vi "LabVIEW FPGA Advanced Interface Tools Installer.vi"() -> ()   [LabVIEW 2010]
panel:
  out "Install Status":string
  in  "Uninstall":bool
  in  "Accept":bool
  out "License":string="Copyright (c) 2011, National Instruments\nAll rights reserved.\n\nRedistribution and use in source and binary forms, with or without modification, are permitted provided that the following conditions are met:\n\no Redistributions of source code must retain the above copyright notice, this list of conditions and the following disclaimer.\no Redistributions in binary form must reproduce the above copyright notice, this list of conditions and the following disclaimer in the documentation and/or other materials provided with the distribution.\no Neither the name of the National Instruments Corporation nor the names of its contributors may be used to endorse or promote products derived from this software without specific prior written permission.\n\nTHIS SOFTWARE IS PROVIDED BY THE COPYRIGHT HOLDERS AND CONTRIBUTORS \"AS IS\" AND ANY EXPRESS OR IMPLIED WARRANTIES, INCLUDING, BUT NOT LIMITED TO, THE IMPLIED WARRANTIES OF MERCHANTABILITY AND FITNESS FOR A PARTICULAR PURPOSE ARE DISCLAIMED. IN NO EVENT SHALL THE COPYRIGHT HOLDER OR CONTRIBUTORS BE LIABLE FOR ANY DIRECT, INDIRECT, INCIDENTAL, SPECIAL, EXEMPLARY, OR CONSEQUENTIAL DAMAGES (INCLUDING, BUT NOT LIMITED TO, PROCUREMENT OF SUBSTITUTE GOODS OR SERVICES; LOSS OF USE, DATA, OR PROFITS; OR BUSINESS INTERRUPTION) HOWEVER CAUSED AND ON ANY THEORY OF LIABILITY, WHETHER IN CONTRACT, STRICT LIABILITY, OR TORT (INCLUDING NEGLIGENCE OR OTHERWISE) ARISING IN ANY WAY OUT OF THE USE OF THIS SOFTWARE, EVEN IF ADVISED OF THE POSSIBILITY OF SUCH DAMAGE."
  in  "Cancel":bool
  in  "Install":bool
  # "LabVIEW FPGA Advanced Interface Tools"
  # "1. Installs FPGA Interfaces to user.lib/_FPGA Interface Advanced Tools.\n2. Installs menus, palettes, and error codes."
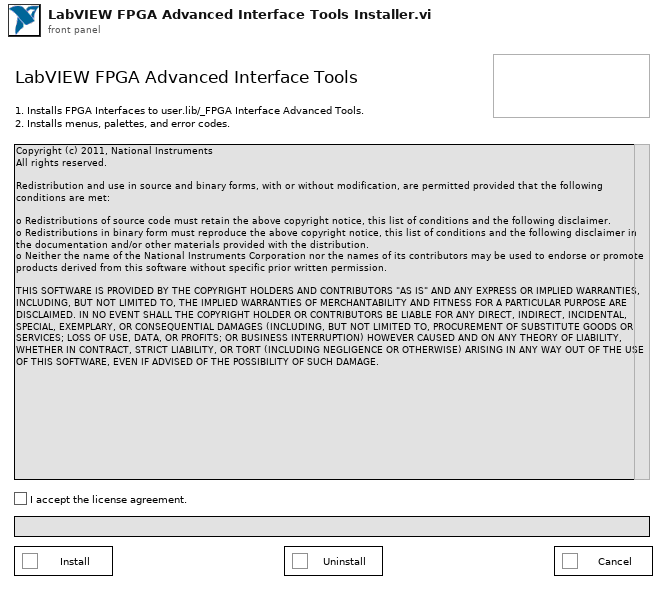
[diagram p1: front panel]
types:
  T1 = enum8{"Enabled", "Disabled", "Disabled and Grayed Out"}
  T2 = enum32{"invalid OS target", "Mac OS", "Windows 3.1", "Windows 95/NT", "Solaris 1", "Solaris 2", "HP-UX", "PowerMAX", "Linux", "Irix", "Rhapsody", "BeOS", "AIX", "OSF1", "VxWorks", "PharLap", "Carbon", "RTX", "Windows x64", "Linux x64"}
  T3 = enum16{"copy labview files", "copy shared files", "copy Xplatform files", "move external linked files to temp", "mass compile", "move temp files to user.lib"}
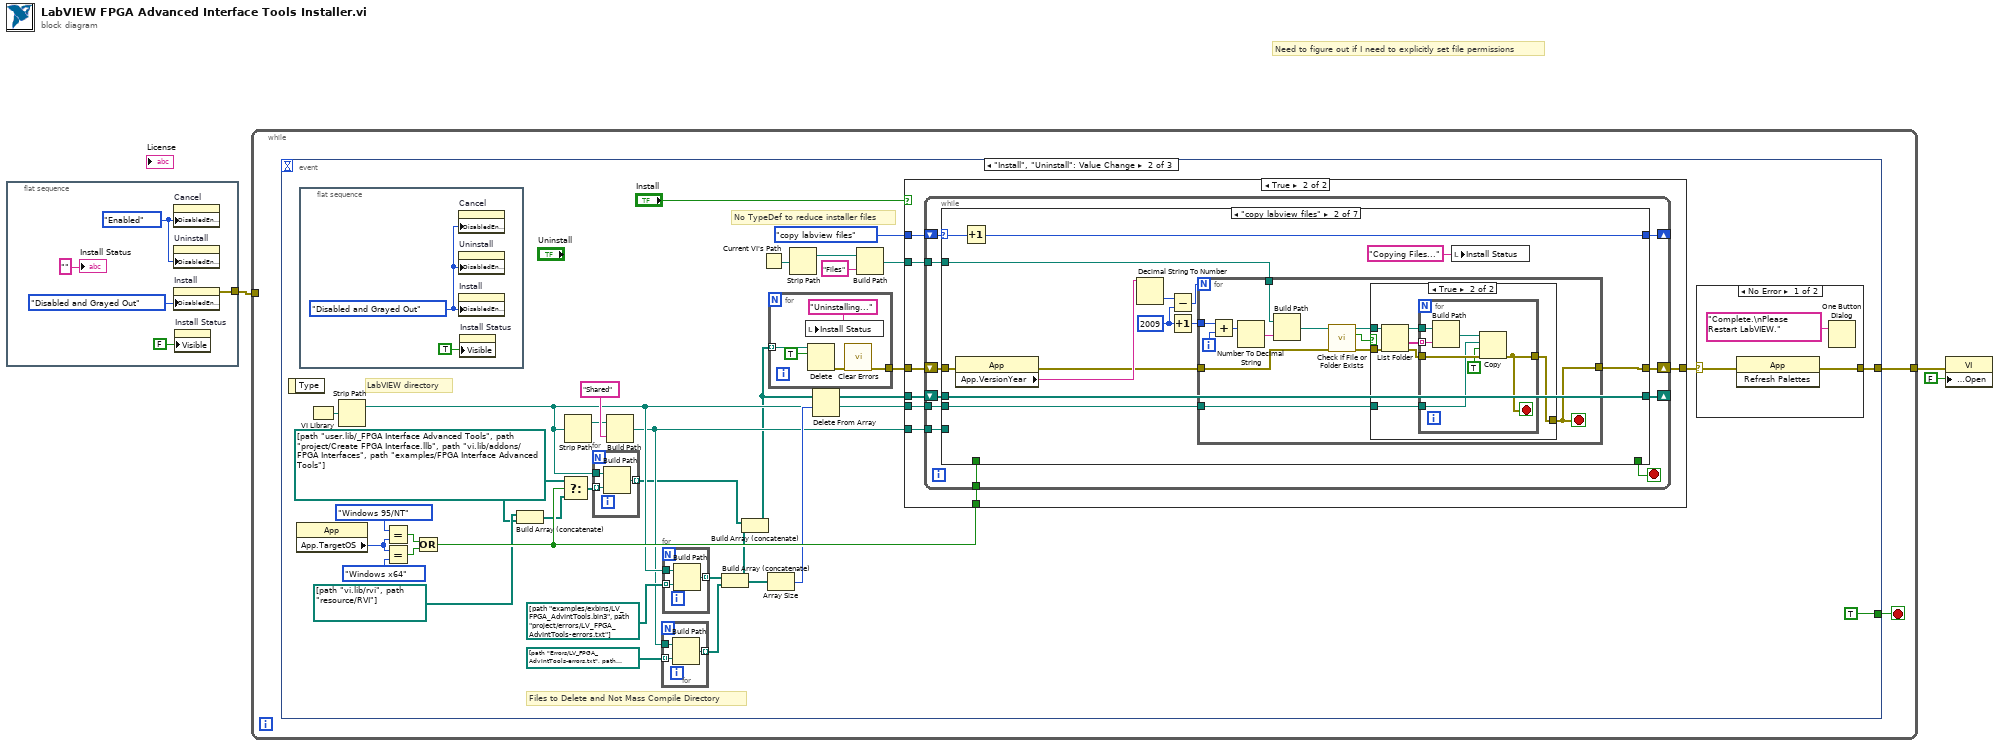
[diagram p0: block diagram]
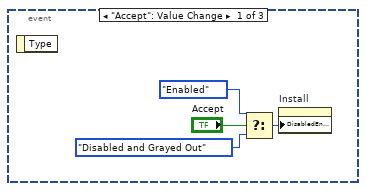
[diagram p2: hidden frame]
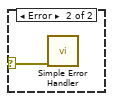
[diagram p3: hidden frame]
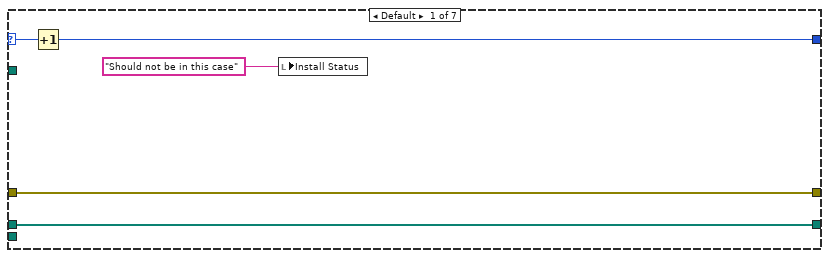
[diagram p5: hidden frame]
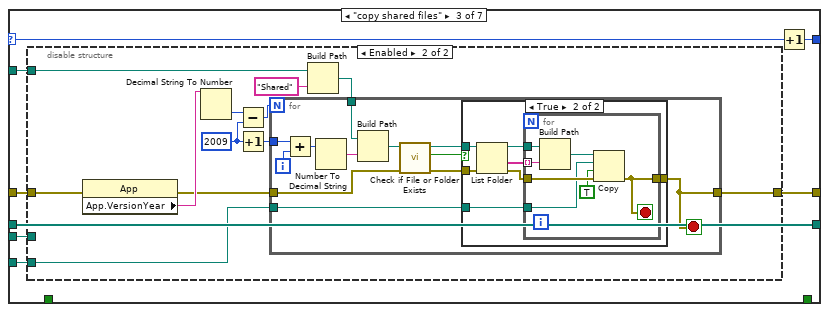
[diagram p7: hidden frame]
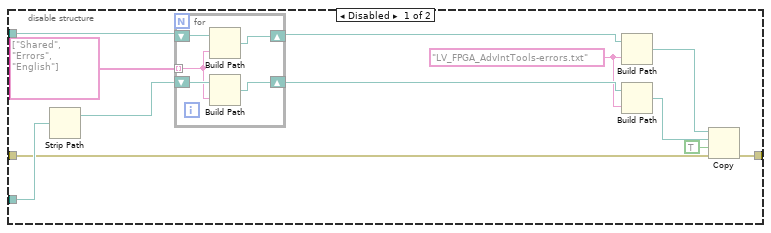
[diagram p8: hidden frame]
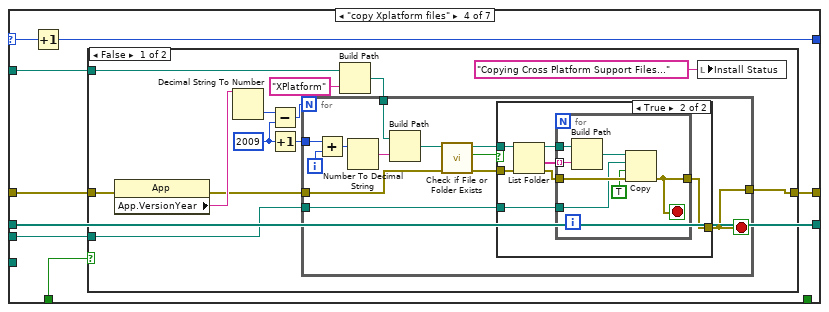
[diagram p10: hidden frame]
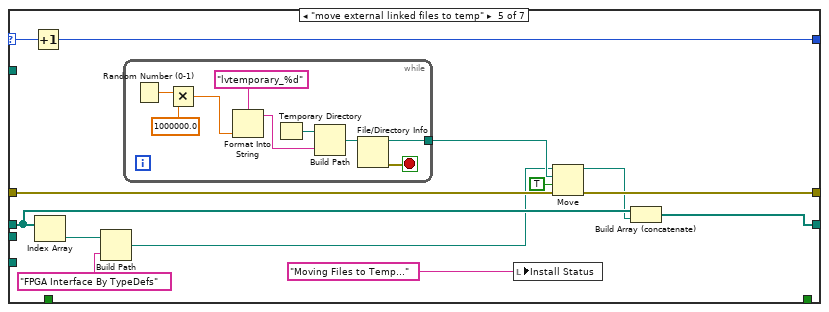
[diagram p13: hidden frame]
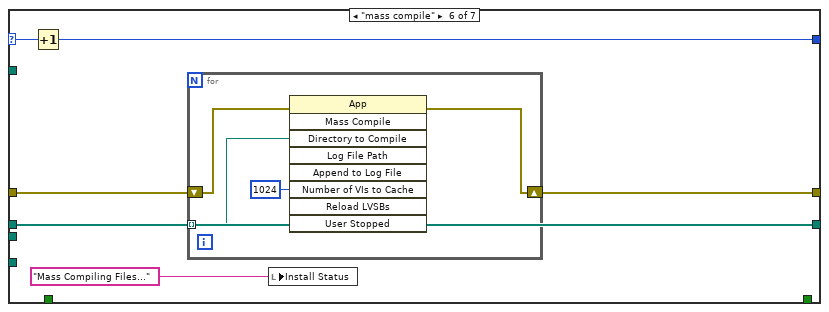
[diagram p14: hidden frame]
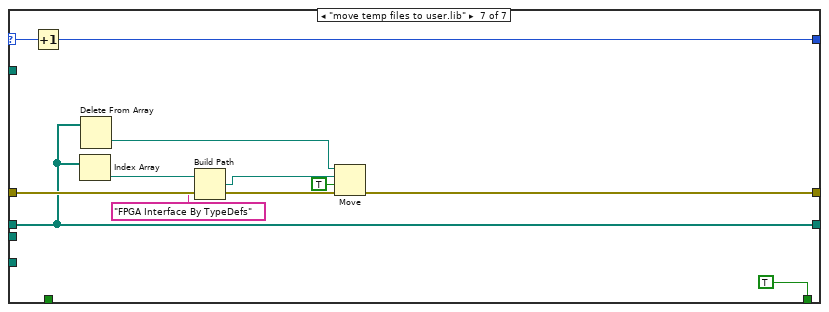
[diagram p15: hidden frame]
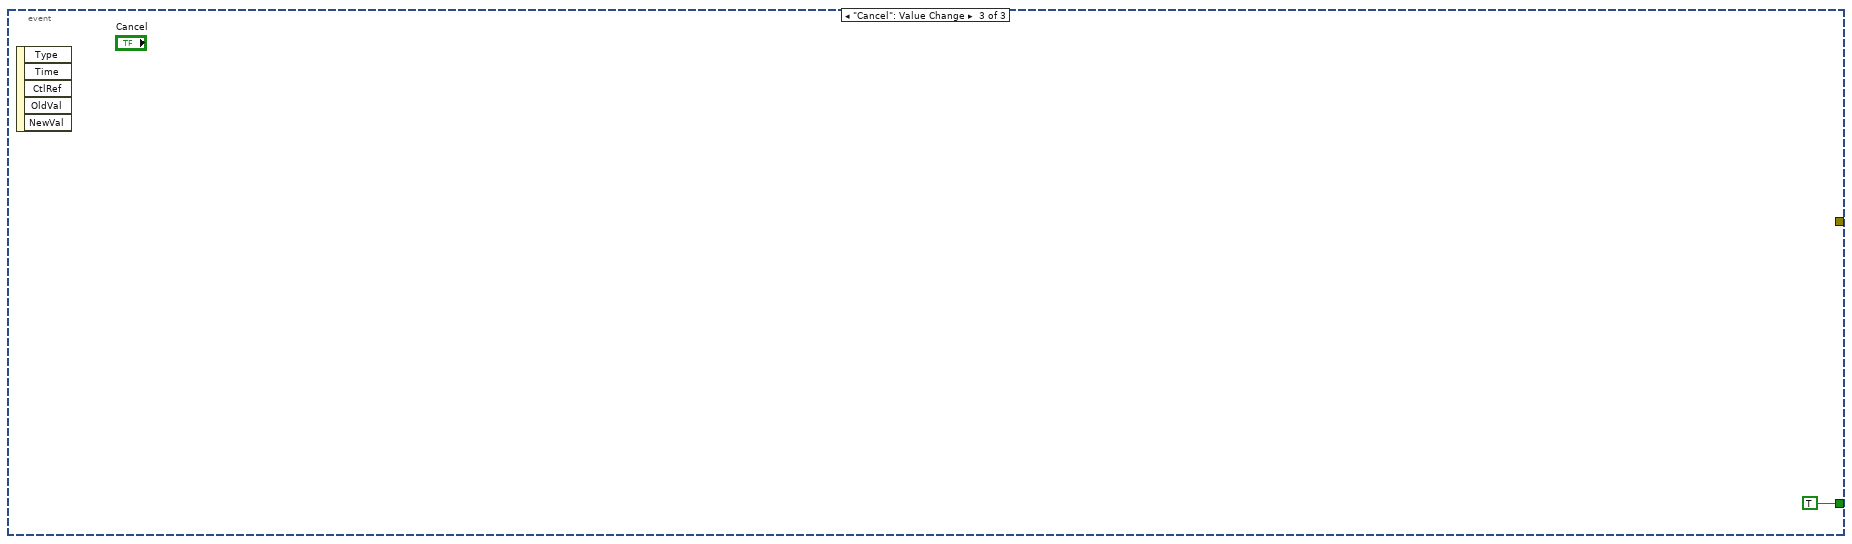
[diagram p16: hidden frame]
diagram:
  # "Need to figure out if I need to explicitly set file permissions"
  n1 = flat-sequence {
    tunnel: [w4] -> w3
    frame #0 {
      w8 = T1."Enabled" ("Disabled")
      n2 = property on="Cancel" class="Bool"("DisabledEnum"=w8) -> ()  [unwired: 2 in, 2 out]
      n3 = property on="Uninstall" class="Bool"("DisabledEnum"=w8) -> ()  [unwired: 2 in, 2 out]
      n4 = property on="Install" class="Bool"("DisabledEnum"=T1."Disabled and Grayed Out" ("Disabled")) -> (error out=w4:errorcluster)  [unwired: 2 in, 1 out]
      n5 = property on="Install Status" class="Str"("Visible"=FALSE) -> ()  [unwired: 2 in, 2 out]
      "Install Status" <- "" ("Install Status")
    }
  }
  n6 = while {
    tunnel: w3 -> [_]
    tunnel: [w9] -> w1
    stop <- w10 stop-if-true
    n7 = event shown="[1] \"Install\", \"Uninstall\": Value Change" {
      selector: _ -> [_ _ _]
      dyn-events: _ -> [_ _ _]
      timeout: _ -> [_ _ _]
      tunnel: [_ TRUE TRUE] -> w10
      tunnel: [_ w38 _] -> w9
      event "Accept": Value Change {
        n8 = event-data() -> ()  [unwired: 1 in, 1 out]
        n9 = Select(t=T1."Enabled" ("Disabled"), s="Accept", f=T1."Disabled and Grayed Out" ("Disabled")) -> (s? t:f=w12:T1)
        n10 = property on="Install" class="Bool"("DisabledEnum"=w12) -> ()  [unwired: 2 in, 2 out]
      }
      event "Install", "Uninstall": Value Change {
        w29 = path[] [path "user.lib/_FPGA Interface Advanced Tools", path "project/Create FPGA Interface.llb", path "vi.lib/addons/FPGA Interfaces", path "examples/FPGA Interface Advanced Tools"]
        # "Files to Delete and Not Mass Compile Directory"
        # "No TypeDef to reduce installer files"
        # "LabVIEW directory"
        n11 = event-data() -> ()  [unwired: 1 in, 1 out]
        n12 = property class="App"() -> ("App.TargetOS"=w33:T2)  [unwired: 2 in, 2 out]
        n13 = flat-sequence {
          frame #0 {
            w290 = T1."Disabled and Grayed Out" ("Disabled")
            n14 = property on="Cancel" class="Bool"("DisabledEnum"=w290) -> ()  [unwired: 2 in, 2 out]
            n15 = property on="Uninstall" class="Bool"("DisabledEnum"=w290) -> ()  [unwired: 2 in, 2 out]
            n16 = property on="Install" class="Bool"("DisabledEnum"=w290) -> ()  [unwired: 2 in, 2 out]
            n17 = property on="Install Status" class="Str"("Visible"=TRUE) -> ()  [unwired: 2 in, 2 out]
          }
        }
        n18 = VI Library() -> (path=w47:path)
        n19 = Strip Path(path=w47) -> (stripped path=w22:path)  [unwired: 1 out]
        n20 = Equal?(x=T2."Windows 95/NT" ("Application:Target:Operating System"), y=w33) -> (x = y?=w37:bool)
        n21 = Equal?(x=w33, y=T2."Windows x64" ("Application:Target:Operating System")) -> (x = y?=w36:bool)
        n22 = Or(x=w37, y=w36) -> (x .or. y?=w32:bool)
        n23 = Build Array (concatenate)(path[] [path "vi.lib/rvi", path "resource/RVI"] ("element"), w29) -> (w31:path[])
        n24 = Select(t=w29, s=w32, f=w31) -> (s? t:f=w26:path[])
        n25 = Strip Path(path=w22) -> (stripped path=w24:path)  [unwired: 1 out]
        n26 = for {
          tunnel: [w57] -> w17 mode=indexing
          tunnel: w26 -> [w56] mode=indexing
          tunnel: w22 -> [w55]
          n27 = Build Path(base path=w55, name or relative path=w56) -> (appended path=w57:path)
        }
        n28 = Build Path(base path=w24, name or relative path="Shared") -> (appended path=w19:path)
        n29 = for {
          tunnel: [w51] -> w20 mode=indexing
          tunnel: path[] [path "Errors/LV_FPGA_AdvIntTools-errors.txt", path "Errors/English/LV_FPGA_AdvIntTools-errors.txt"] ("element") -> [w50] mode=indexing
          tunnel: w19 -> [w49]
          n30 = Build Path(base path=w49, name or relative path=w50) -> (appended path=w51:path)
        }
        n31 = for {
          tunnel: [w54] -> w21 mode=indexing
          tunnel: path[] [path "examples/exbins/LV_FPGA_AdvIntTools.bin3", path "project/errors/LV_FPGA_AdvIntTools-errors.txt"] ("element") -> [w53] mode=indexing
          tunnel: w22 -> [w52]
          n32 = Build Path(base path=w52, name or relative path=w53) -> (appended path=w54:path)
        }
        n33 = Build Array (concatenate)(w21, w20) -> (w18:path[])
        n34 = Build Array (concatenate)(w17, w18) -> (w15:path[])
        n35 = Current VI's Path() -> (path=w46:path)
        n36 = Array Size(array=w18) -> (size(s)=w27:i32)
        n37 = for {
          tunnel: w15 -> [w284] mode=indexing
          tunnel: [w285] -> w40
          n38 = local write "Install Status"("Uninstalling..." ("Install Status")) -> ()
          n39 = Delete(path (use dialog)=w284, entire hierarchy (F)=TRUE) -> (error out=w286:errorcluster)  [unwired: 3 in, 2 out]
          n40 = call <vilib>:"Clear Errors.vi"("error in (no error)"=w286) -> ("error out"=w285:errorcluster)  [unwired: 6 in]
        }
        n41 = Strip Path(path=w46) -> (stripped path=w45:path)  [unwired: 1 out]
        n42 = Delete From Array(array=w15, length=w27) -> (array with subset deleted=w28:path[])  [unwired: 1 in, 1 out]
        n43 = Build Path(base path=w45, name or relative path="Files") -> (appended path=w41:path)
        n44 = case shown="True" "Install" {
          tunnel: T3."copy labview files" -> [_ w70]
          tunnel: w41 -> [_ w69]
          tunnel: w40 -> [w62 w68]
          tunnel: w22 -> [_ w67]
          tunnel: w28 -> [_ w66]
          tunnel: [w62 w65] -> w39
          tunnel: w32 -> [_ w64]
          tunnel: w19 -> [_ w63]
          frame False {
          }
          frame True {
            n45 = while {
              shift-right: [w80] -> _
              shift-left: w70 -> [w81]
              tunnel: w69 -> [w78]
              shift-right: [w75] -> w65
              shift-left: w68 -> [w77]
              tunnel: w67 -> [w76]
              shift-right: [w73] -> _
              shift-left: w66 -> [w74]
              tunnel: w64 -> [w72]
              tunnel: w63 -> [w71]
              stop <- w79 stop-if-true
              n46 = case shown="\"copy labview files\"" w81 {
                selector: w81 -> [w86 w100 w130 w199 w253 w268 w283]
                tunnel: [w85 w99 w129 w198 w252 w267 w282] -> w80
                tunnel: [_ _ _ _ _ _ TRUE] -> w79
                tunnel: w78 -> [_ w92 w134 w197 _ _ _]
                tunnel: w77 -> [w82 w98 w132 w194 w246 w265 w279]
                tunnel: w76 -> [_ w91 w133 w196 _ _ _]
                tunnel: [w82 w87 w131 w195 w244 w264 w278] -> w75
                tunnel: w74 -> [w83 w89 w135 w192 w251 w263 w274]
                tunnel: [w83 w89 w135 w192 w242 w263 w274] -> w73
                tunnel: w72 -> [_ _ _ w193 _ _ _]
                tunnel: w71 -> [_ _ w128 _ _ _ _]
                frame Default {
                  n47 = Increment(x=w86) -> (x+1=w85:T3)
                  n48 = local write "Install Status"("Should not be in this case" ("Install Status")) -> ()
                }
                frame "copy labview files" {
                  w94 = 2009 ("y")
                  n49 = property class="App"(error in=w98) -> (error out=w88:errorcluster, "App.VersionYear"=w97:string)  [unwired: 1 in, 1 out]
                  n50 = Increment(x=w100) -> (x+1=w99:T3)
                  n51 = Decimal String To Number(string=w97) -> (number=w96:i32)  [unwired: 2 in, 1 out]
                  n52 = Subtract(x=w96, y=w94) -> (x-y=w95:i32)
                  n53 = Increment(x=w94) -> (x+1=w93:i32)
                  n54 = for {
                    N: w95 -> [_]
                    tunnel: w93 -> [w112]
                    tunnel: w92 -> [w108]
                    tunnel: w91 -> [w107]
                    tunnel: w88 -> [w106]
                    tunnel: [w105] -> w87
                    i -> [w111]
                    stop <- w105 stop-if-true
                    n55 = Add(x=w112, y=w111) -> (x+y=w110:i32)
                    n56 = Number To Decimal String(number=w110) -> (decimal integer string=w109:string)  [unwired: 1 in]
                    n57 = Build Path(base path=w108, name or relative path=w109) -> (appended path=w103:path)
                    n58 = call <vilib>:"Check if File or Folder Exists.vi"("error in (no error)"=w106, "path"=w103) -> ("error out"=w104:errorcluster, "file or folder exists?"=w101:bool, "dup path"=w102:path)  [unwired: 7 in]
                    n59 = case shown="True" w101 {
                      tunnel: w102 -> [_ w117]
                      tunnel: w107 -> [_ w116]
                      tunnel: w104 -> [w113 w115]
                      tunnel: [w113 w114] -> w105
                      frame False {
                      }
                      frame True {
                        n60 = List Folder(path=w117, error in=w115) -> (path out=w119:path, folder names=w118:string[], error out=w120:errorcluster)  [unwired: 2 in, 1 out]
                        n61 = for {
                          tunnel: w118 -> [w126] mode=indexing
                          tunnel: w119 -> [w127]
                          tunnel: w116 -> [w122]
                          tunnel: w120 -> [w124]
                          tunnel: [w121] -> w114
                          stop <- w121 stop-if-true
                          n62 = Build Path(base path=w127, name or relative path=w126) -> (appended path=w125:path)
                          n63 = Copy(8:w124, 9:TRUE ("overwrite (F)"), 10:w122, 11:w125) -> (0:w121:errorcluster)  [unwired: 1 in, 2 out]
                        }
                      }
                    }
                  }
                  n64 = local write "Install Status"("Copying Files..." ("Install Status")) -> ()
                }
                frame "copy shared files" {
                  n65 = disable-structure shown="Enabled" {
                    disable-tunnel: w134 -> [w147 w155]
                    disable-tunnel: w133 -> [w146 _]
                    disable-tunnel: w132 -> [w143 w156]
                    disable-tunnel: [w137 w153] -> w131
                    disable-tunnel: w128 -> [_ w154]
                    frame Disabled {
                      w141 = "LV_FPGA_AdvIntTools-errors.txt" ("name or relative path")
                      n66 = Strip Path(path=w146) -> (stripped path=w145:path)  [unwired: 1 out]
                      n67 = for {
                        tunnel: string[] ["Shared", "Errors", "English"] -> [w150] mode=indexing
                        shift-right: [w149] -> w144
                        shift-left: w147 -> [w152]
                        shift-right: [w148] -> w142
                        shift-left: w145 -> [w151]
                        n68 = Build Path(base path=w152, name or relative path=w150) -> (appended path=w149:path)
                        n69 = Build Path(base path=w151, name or relative path=w150) -> (appended path=w148:path)
                      }
                      n70 = Build Path(base path=w144, name or relative path=w141) -> (appended path=w139:path)
                      n71 = Build Path(base path=w142, name or relative path=w141) -> (appended path=w140:path)
                      n72 = Copy(8:w143, 9:TRUE ("overwrite (F)"), 10:w140, 11:w139) -> (0:w137:errorcluster)  [unwired: 1 in, 2 out]
                    }
                    frame Enabled {
                      w162 = 2009 ("y")
                      n73 = property class="App"(error in=w156) -> (error out=w157:errorcluster, "App.VersionYear"=w158:string)  [unwired: 1 in, 1 out]
                      n74 = Decimal String To Number(string=w158) -> (number=w164:i32)  [unwired: 2 in, 1 out]
                      n75 = Subtract(x=w164, y=w162) -> (x-y=w163:i32)
                      n76 = Increment(x=w162) -> (x+1=w161:i32)
                      n77 = Build Path(base path=w155, name or relative path="Shared") -> (appended path=w160:path)
                      n78 = for {
                        N: w163 -> [_]
                        tunnel: w161 -> [w176]
                        tunnel: w160 -> [w172]
                        tunnel: w154 -> [w171]
                        tunnel: w157 -> [w170]
                        tunnel: [w169] -> w153
                        i -> [w175]
                        stop <- w169 stop-if-true
                        n79 = Add(x=w176, y=w175) -> (x+y=w174:i32)
                        n80 = Number To Decimal String(number=w174) -> (decimal integer string=w173:string)  [unwired: 1 in]
                        n81 = Build Path(base path=w172, name or relative path=w173) -> (appended path=w167:path)
                        n82 = call <vilib>:"Check if File or Folder Exists.vi"("error in (no error)"=w170, "path"=w167) -> ("error out"=w168:errorcluster, "file or folder exists?"=w165:bool, "dup path"=w166:path)  [unwired: 7 in]
                        n83 = case shown="True" w165 {
                          tunnel: w171 -> [_ w181]
                          tunnel: [w177 w180] -> w169
                          tunnel: w168 -> [w177 w179]
                          tunnel: w166 -> [_ w178]
                          frame False {
                          }
                          frame True {
                            n84 = List Folder(path=w178, error in=w179) -> (path out=w183:path, folder names=w182:string[], error out=w184:errorcluster)  [unwired: 2 in, 1 out]
                            n85 = for {
                              tunnel: w182 -> [w190] mode=indexing
                              tunnel: w183 -> [w191]
                              tunnel: w181 -> [w186]
                              tunnel: w184 -> [w188]
                              tunnel: [w185] -> w180
                              stop <- w185 stop-if-true
                              n86 = Build Path(base path=w191, name or relative path=w190) -> (appended path=w189:path)
                              n87 = Copy(8:w188, 9:TRUE ("overwrite (F)"), 10:w186, 11:w189) -> (0:w185:errorcluster)  [unwired: 1 in, 2 out]
                            }
                          }
                        }
                      }
                    }
                  }
                  n88 = Increment(x=w130) -> (x+1=w129:T3)
                }
                frame "copy Xplatform files" {
                  n89 = Increment(x=w199) -> (x+1=w198:T3)
                  n90 = case shown="False" w193 {
                    tunnel: w197 -> [w206 _]
                    tunnel: w196 -> [w208 _]
                    tunnel: w194 -> [w203 w240]
                    tunnel: [w200 w240] -> w195
                    frame False {
                      w210 = 2009 ("y")
                      n91 = property class="App"(error in=w203) -> (error out=w201:errorcluster, "App.VersionYear"=w202:string)  [unwired: 1 in, 1 out]
                      n92 = Decimal String To Number(string=w202) -> (number=w212:i32)  [unwired: 2 in, 1 out]
                      n93 = Subtract(x=w212, y=w210) -> (x-y=w211:i32)
                      n94 = Increment(x=w210) -> (x+1=w209:i32)
                      n95 = Build Path(base path=w206, name or relative path="XPlatform") -> (appended path=w205:path)
                      n96 = for {
                        N: w211 -> [_]
                        tunnel: w209 -> [w224]
                        tunnel: w205 -> [w220]
                        tunnel: w208 -> [w219]
                        tunnel: w201 -> [w218]
                        tunnel: [w214] -> w200
                        i -> [w223]
                        stop <- w214 stop-if-true
                        n97 = Add(x=w224, y=w223) -> (x+y=w222:i32)
                        n98 = Number To Decimal String(number=w222) -> (decimal integer string=w221:string)  [unwired: 1 in]
                        n99 = Build Path(base path=w220, name or relative path=w221) -> (appended path=w216:path)
                        n100 = call <vilib>:"Check if File or Folder Exists.vi"("error in (no error)"=w218, "path"=w216) -> ("error out"=w217:errorcluster, "file or folder exists?"=w213:bool, "dup path"=w215:path)  [unwired: 7 in]
                        n101 = case shown="True" w213 {
                          tunnel: w219 -> [_ w229]
                          tunnel: w217 -> [w225 w228]
                          tunnel: w215 -> [_ w227]
                          tunnel: [w225 w226] -> w214
                          frame False {
                          }
                          frame True {
                            n102 = List Folder(path=w227, error in=w228) -> (path out=w231:path, folder names=w230:string[], error out=w232:errorcluster)  [unwired: 2 in, 1 out]
                            n103 = for {
                              tunnel: w230 -> [w238] mode=indexing
                              tunnel: w231 -> [w239]
                              tunnel: w229 -> [w234]
                              tunnel: w232 -> [w236]
                              tunnel: [w233] -> w226
                              stop <- w233 stop-if-true
                              n104 = Build Path(base path=w239, name or relative path=w238) -> (appended path=w237:path)
                              n105 = Copy(8:w236, 9:TRUE ("overwrite (F)"), 10:w234, 11:w237) -> (0:w233:errorcluster)  [unwired: 1 in, 2 out]
                            }
                          }
                        }
                      }
                      n106 = local write "Install Status"("Copying Cross Platform Support Files..." ("Install Status")) -> ()
                    }
                    frame True {
                    }
                  }
                }
                frame "move external linked files to temp" {
                  n107 = Increment(x=w253) -> (x+1=w252:T3)
                  n108 = Index Array(array=w251) -> (element=w250:path)  [unwired: 1 in]
                  n109 = Build Path(base path=w250, name or relative path="FPGA Interface By TypeDefs") -> (appended path=w245:path)
                  n110 = while {
                    tunnel: [w254] -> w247
                    stop <- w255 stop-if-true
                    n111 = Random Number (0-1)() -> (number: 0 to 1=w262:dbl)
                    n112 = Multiply(x=w262, y=1000000.0) -> (x*y=w259:dbl)
                    n113 = Format Into String(format string="lvtemporary_%d", w259) -> (resulting string=w258:string)  [unwired: 2 in, 1 out]
                    n114 = Temporary Directory() -> (w257:path)
                    n115 = Build Path(base path=w257, name or relative path=w258) -> (appended path=w256:path)
                    n116 = File/Directory Info(path=w256) -> (path out=w254:path, error out=w255:errorcluster)  [unwired: 1 in, 5 out]
                  }
                  n117 = local write "Install Status"("Moving Files to Temp..." ("Install Status")) -> ()
                  n118 = Move(source path=w245, error in=w246, 9:TRUE ("overwrite (F)"), 10:w247) -> (error out=w244:errorcluster, 3:w241:path)  [unwired: 1 in, 1 out]
                  n119 = Build Array (concatenate)(w251, w241) -> (w242:path[])
                }
                frame "mass compile" {
                  n120 = Increment(x=w268) -> (x+1=w267:T3)
                  n121 = for {
                    shift-right: [w271] -> w264
                    shift-left: w265 -> [w272]
                    tunnel: w263 -> [w270] mode=indexing
                    n122 = invoke class="App" method="Mass Compile"(error in=w272, "Directory to Compile"=w270, "Number of VIs to Cache"=u32 1024) -> (error out=w271:errorcluster)  [unwired: 6 in, 8 out]
                  }
                  n123 = local write "Install Status"("Mass Compiling Files..." ("Install Status")) -> ()
                }
                frame "move temp files to user.lib" {
                  n124 = Increment(x=w283) -> (x+1=w282:T3)
                  n125 = Index Array(array=w274) -> (element=w275:path)  [unwired: 1 in]
                  n126 = Delete From Array(array=w274) -> (deleted portion=w273:path)  [unwired: 2 in, 1 out]
                  n127 = Build Path(base path=w275, name or relative path="FPGA Interface By TypeDefs") -> (appended path=w276:path)
                  n128 = Move(source path=w273, error in=w279, 9:TRUE ("overwrite (F)"), 10:w276) -> (error out=w278:errorcluster)  [unwired: 1 in, 2 out]
                }
              }
            }
          }
        }
        n129 = case shown="No Error" w39 {
          selector: w39 -> [w59 w61]
          tunnel: [w58 _] -> w38
          frame No Error {
            n130 = invoke class="App" method="Refresh Palettes"(error in=w59) -> (error out=w58:errorcluster)  [unwired: 2 in, 2 out]
            n131 = One Button Dialog(message="Complete.\nPlease Restart LabVIEW." ("Install Status")) -> ()  [unwired: 1 in, 1 out]
          }
          frame Error {
            n132 = call <vilib>:"Simple Error Handler.vi"("error in (no error)"=w61) -> ()  [unwired: 4 in, 5 out]
          }
        }
      }
      event "Cancel": Value Change {
        n133 = event-data() -> ()  [unwired: 1 in, 5 out]
      }
    }
  }
  n134 = property class="VI"(error in=w1, "Front Panel.Open"=FALSE ("Front Panel Window:Open")) -> ()  [unwired: 1 in, 2 out]
